vi "GraphView_Read.vi"(8 "error in (no error)":errorcluster) -> (0 "error out":errorcluster)   [LabVIEW 2019]
uses:
  <vilib>/Analysis/3filter.llb/Filter Passband Type.ctl
  _ctrl/rw.ctl
  <vilib>/Analysis/3filter.llb/Butterworth Filter (DBL).vi
  <vilib>/Analysis/NI_AALBase.lvlib
panel:
  in  "order":i32=2
  in  "Return":bool
  in  "low cutoff freq: fl":dbl=0.12500000000000006 format="%0.4f"
  in  "high cutoff freq: fh":dbl=0.45000000000000007 format="%0.2f"
  in  "sampling freq: fs":dbl=1.0 format="%0.2f"
  in  "Filter":bool
  in  "filter type":T1
  in  "Exit":bool
  out "Waveform_DLM5038":cluster{"l":dbl, "dt":dbl, "Y":dbl[][]}(graph)
  # "DL950 Waveform"
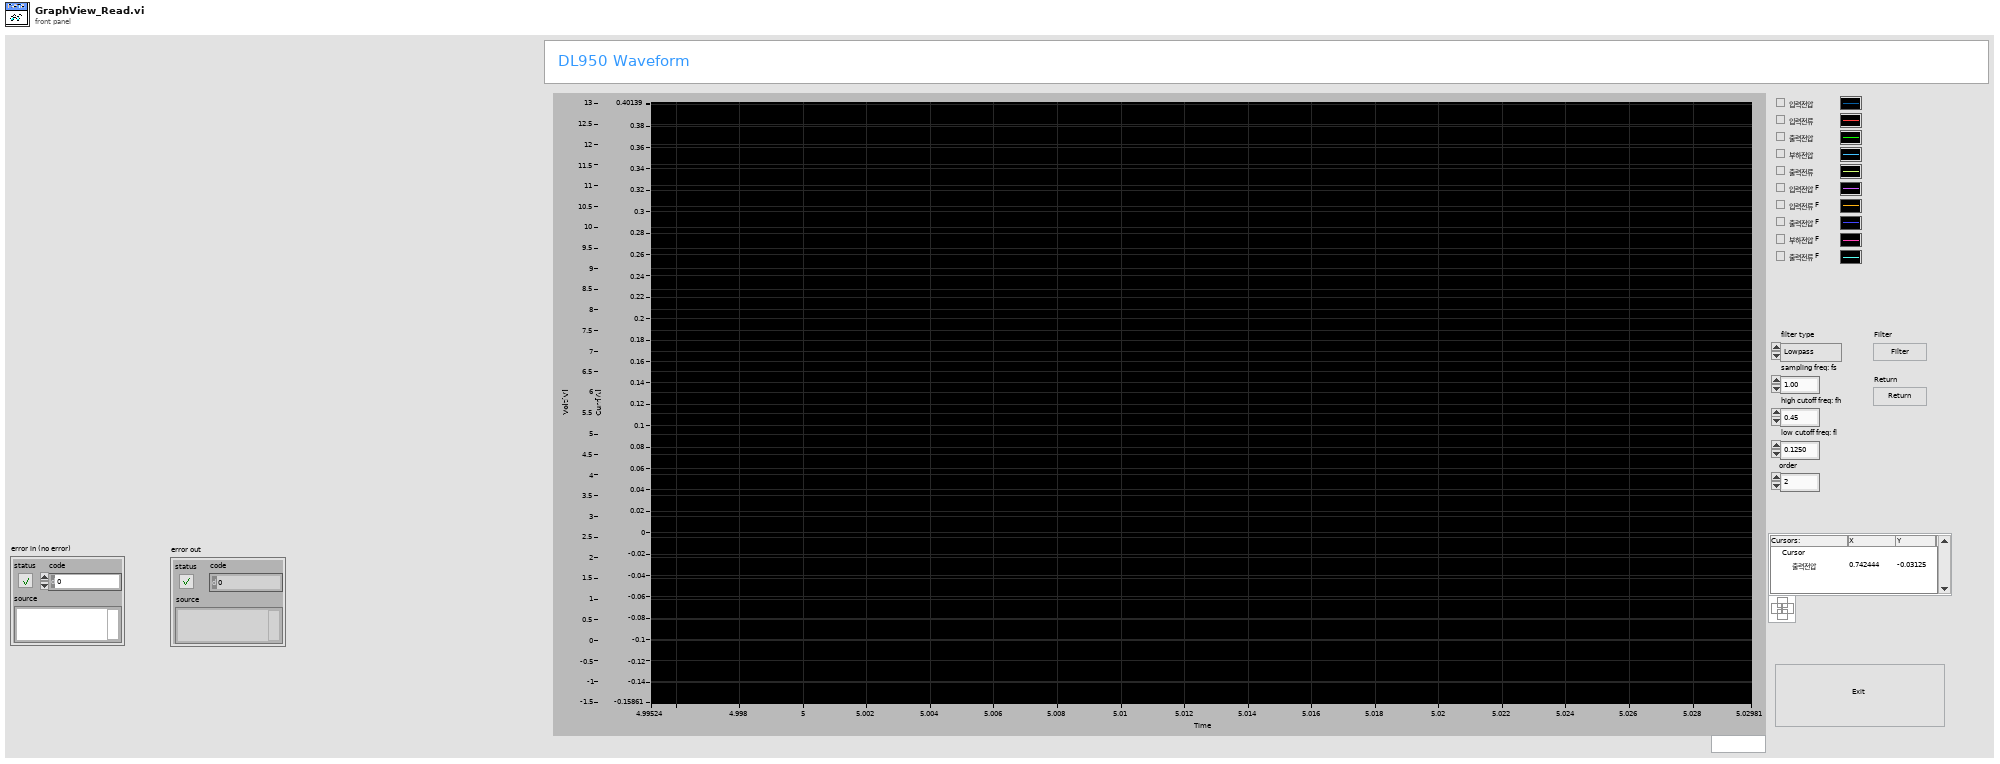
[diagram p1: front panel]
types:
  T1 = typedef "NI_AALBase.lvlib/Filter Passband Type.ctl" = enum32{"Lowpass", "Highpass", "Bandpass", "Bandstop"}
  T2 = typedef "rw.ctl" = enum16{"read", "write"}
  T3 = typedef "DL950_wfms.ctl" = cluster{"wfms":waveform(dbl)[], "Waveform_2":cluster{"t0":dbl, "dt":dbl, "Y":dbl[][]}, "items":dbl[][], "da950_array":dbl[]}
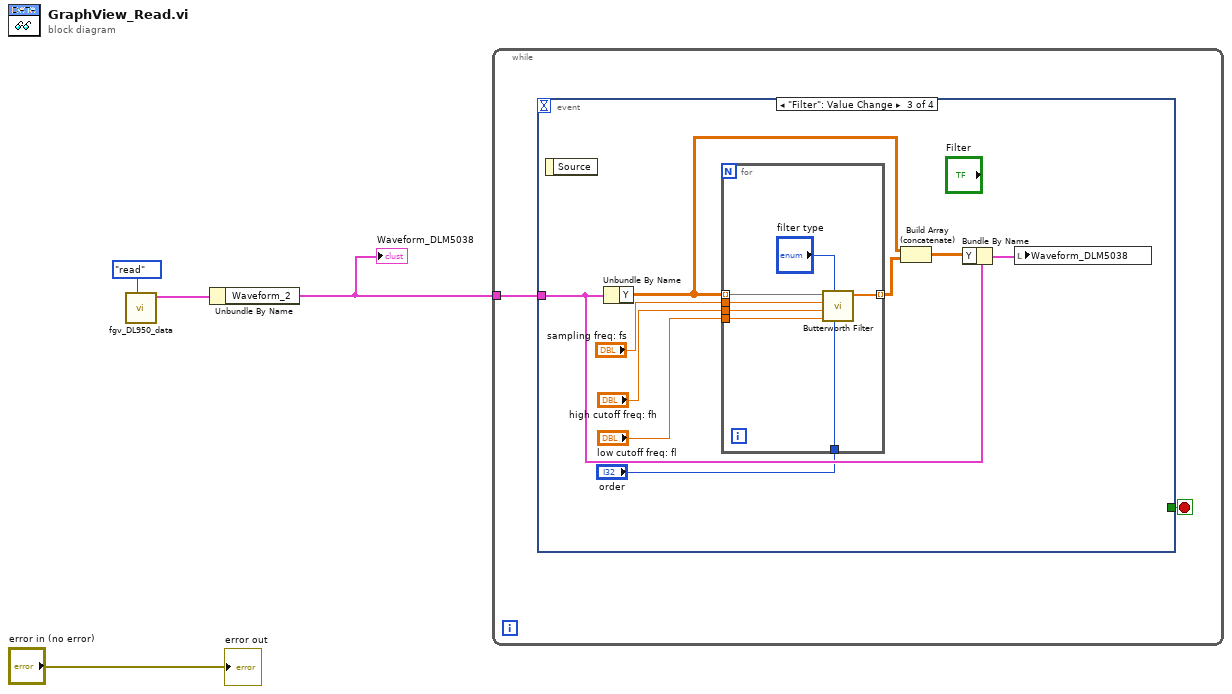
[diagram p0: block diagram]
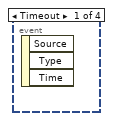
[diagram p2: hidden frame]
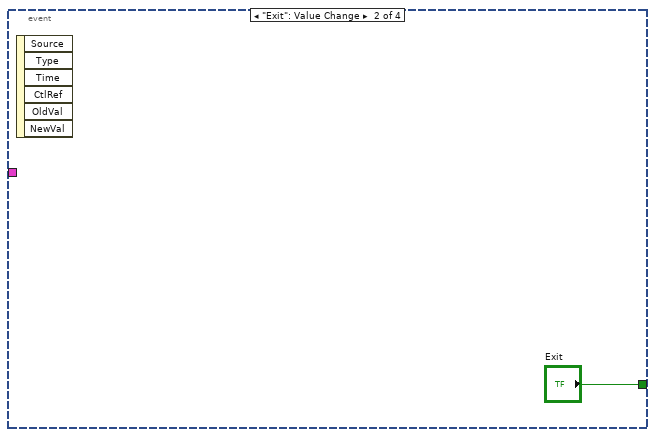
[diagram p3: hidden frame]
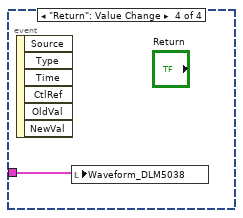
[diagram p4: hidden frame]
diagram:
  n1 = call "fgv_DL950_data.vi"("cmd"=rw."read") -> ("DL950 wfm 2"=w2:T3)  [unwired: 9 in, 1 out]
  n2 = Unbundle By Name(w2) -> ("Waveform_2"=w1:cluster{"t0":dbl, "dt":dbl, "Y":dbl[][]})
  "Waveform_DLM5038" <- w1
  n3 = while {
    tunnel: w1 -> [w5]
    stop <- w6 stop-if-true
    n4 = event shown="[2] \"Filter\": Value Change" {
      selector: _ -> [_ _ _ _]
      dyn-events: _ -> [_ _ _ _]
      timeout: _ -> [_ _ _ _]
      tunnel: [_ "Exit" _ _] -> w6
      tunnel: w5 -> [_ _ w13 w24]
      event Timeout {
        n5 = event-data() -> ()  [unwired: 1 in, 3 out]
      }
      event "Exit": Value Change {
        n6 = event-data() -> ()  [unwired: 1 in, 6 out]
      }
      event "Filter": Value Change {
        n7 = event-data() -> ()  [unwired: 1 in, 1 out]
        n8 = Unbundle By Name(w13) -> ("Y"=w11:dbl[][])
        n9 = for {
          tunnel: w11 -> [w22] mode=indexing
          tunnel: "high cutoff freq: fh" -> [w21]
          tunnel: "sampling freq: fs" -> [w20]
          tunnel: "low cutoff freq: fl" -> [w19]
          tunnel: [w18] -> w10 mode=indexing
          tunnel: "order" -> [w17]
          n10 = call-poly <vilib>:"Butterworth Filter.vi"("order"=w17, "filter type"="filter type", "low cutoff freq: fl"=w19, "high cutoff freq: fh"=w21, "sampling freq: fs"=w20, "X"=w22) -> ("Filtered X"=w18:dbl[])  [unwired: 2 in, 1 out]
        }
        n11 = Build Array (concatenate)(w11, w10) -> (w9:dbl[][])
        n12 = Bundle By Name(cluster=w13, "Y"=w9) -> (w12:cluster{"t0":dbl, "dt":dbl, "Y":dbl[][]})
        n13 = local write "Waveform_DLM5038"(w12) -> ()
      }
      event "Return": Value Change {
        n14 = event-data() -> ()  [unwired: 1 in, 6 out]
        n15 = local write "Waveform_DLM5038"(w24) -> ()
      }
    }
  }
  "error out" <- "error in (no error)"
